vi "Request Motor State Update.vi"(8 "error in (no error)":errorcluster, 11 "Elevator in":refnum<class "Elevator.lvclass">) -> (0 "error out":errorcluster, 3 "Elevator out":refnum<class "Elevator.lvclass">)   [LabVIEW 2014, in "Elevator.lvlib" / "Elevator.lvclass"]
uses:
  Elevator.lvclass
  Elevator Messages/Current Motors with Encoder State Msg/Current Motors with Encoder State Msg.lvclass
  <vilib>/ActorFramework/Actor/Actor.lvclass/Actor.ctl
  <vilib>/ActorFramework/Message Enqueuer/Message Enqueuer.lvclass/Message Enqueuer.ctl
  Elevator.lvclass/Elevator.ctl
  Motor with Encoders/Motors with Encoders Messages/Request Motors with Encoders State Msg/Request Motors with Encoders State Msg.lvclass/Request Motors with Encoders State Msg.ctl
  <vilib>/ActorFramework/Message Enqueuer/Init from Existing Queue.vi
  <vilib>/ActorFramework/Message Enqueuer/Enqueue.vi
  <vilib>/ActorFramework/Message Priority Queue/Priority Enqueue.vi
  <vilib>/ActorFramework/Message Enqueuer/Message Enqueuer.lvclass
  Motor with Encoders/Motors with Encoders Messages/Request Motors with Encoders State Msg/Request Motors with Encoders State Msg.lvclass
  <vilib>/ActorFramework/Actor/Actor.lvclass
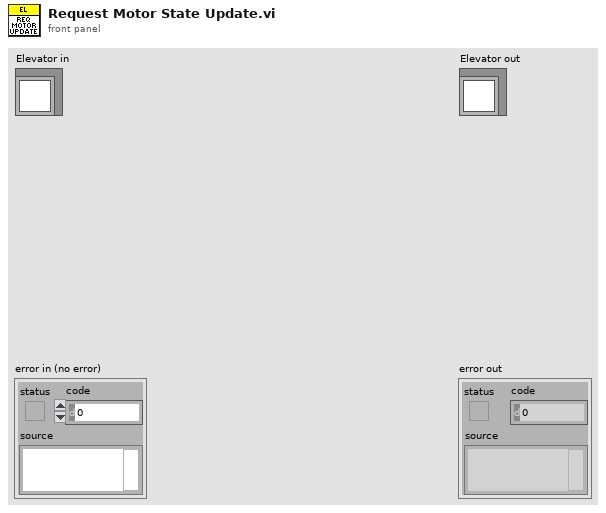
[diagram p1: front panel]
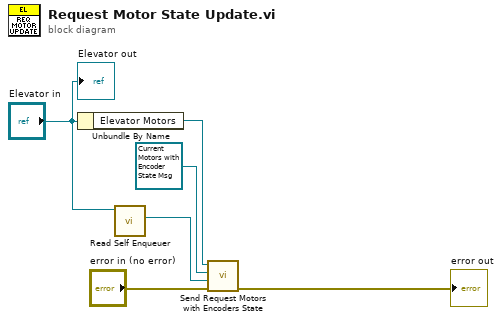
[diagram p0: block diagram]
diagram:
  n1 = Unbundle By Name("Elevator in") -> ("Elevator Motors"=w6:refnum<class "Message Enqueuer.lvclass">)
  n2 = call <vilib>:"Read Self Enqueuer.vi"("Actor"="Elevator in") -> ("Self Enqueuer"=w3:refnum<class "Message Enqueuer.lvclass">)  [unwired: 10 in]
  n3 = call "Send Request Motors with Encoders State.vi"("error in (no error)"="error in (no error)", "Requestor Queue"=w3, "Current State Msg"=refnum<class "Current Motors with Encoder State Msg.lvclass"> refnum ("Elevator.lvlib:Current Motors with Encoder State Msg.lvclass"), "Message Enqueuer"=w6) -> ("error out"=→"error out":errorcluster)  [unwired: 6 in, 1 out]
  "Elevator out" <- "Elevator in"
